vi "Periodic Tasks.vi"(8 "error in":errorcluster) -> ()   [LabVIEW 2017]
doc: "This VI runs in parallel to other tasks. It can contain as many user-defined periodic loops as you need. These can carry out PID or other sorts of timed response."
uses:
  <vilib>/Rock Robotics/WPI/DriverStation/WPI_DriverStationRobotMode2.ctl
  <vilib>/Rock Robotics/WPI/Utilities/WPI_GetSetVariantRefNum.vi
  Robot Global Data.vi
  <vilib>/Rock Robotics/WPI/RobotDrive/WPI_RobotDriveArcadeDrive_Standard(NoSaturation).vi
  <vilib>/Rock Robotics/Network Tables/NT Write Numeric Array.vi
  <vilib>/Rock Robotics/Network Tables/NT Write Number.vi
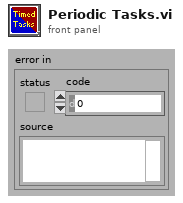
[diagram p1: front panel]
types:
  T1 = typedef "WPI_JoystickDevRef.ctl" = cluster{"Device":T2}
  T2 = typedef "WPI_JoystickDeviceEnum.ctl" = enum16{"USB 0", "USB 1", "USB 2", "USB 3", "USB 4", "USB 5"}
  T3 = typedef "WPI_RobotDriveDevRef.ctl" = cluster{"DevStatus":errorcluster, "Motors[]":T4[], "Square Inputs":bool, "Max Output":dbl}
  T4 = typedef "WPI_MotorControlDeviceRef.ctl" = cluster{"DeviceStatus":errorcluster, "Type":T5, "PWM":cluster{"PWM Channel":T6, "DeadBand":T7}, "CAN":cluster{"Device Number":u8, "SetOutput VI Ref":variant, "GetOutput VI Ref":variant, "Enable VI Ref":variant, "Disable VI Ref":variant, "Data":variant}, "Invert":bool, "DIO PWM":cluster{"PWM \"Enable\" Channel":T6, "DIOChannel":T8, "PWM Rate":dbl}}
  T5 = typedef "WPI_MotorControlType.ctl" = enum16{"PWM", "CAN", "DIO PWM"}
  T6 = typedef "FPGA_DIOPWMChannel.ctl" = enum8{"PWM 0", "PWM 1", "PWM 2", "PWM 3", "PWM 4", "PWM 5", "PWM 6", "PWM 7", "PWM 8", "PWM 9", "PWM MXP 0", "PWM MXP 1", "PWM MXP 2", "PWM MXP 3", "PWM MXP 4", "PWM MXP 5", "PWM MXP 6", "PWM MXP 7", "PWM MXP 8", "PWM MXP 9", "Invalid"}
  T7 = typedef "WPI_PWMDeadband.ctl" = cluster{"Name":string, "maxPositivePwm":i32, "minPositivePwm":i32, "centerPwm":i32, "maxNegativePwm":i32, "minNegativePwm":i32, "angularRange":u16}
  T8 = typedef "FPGA_DIOChannel.ctl" = enum8{"DIO 0", "DIO 1", "DIO 2", "DIO 3", "DIO 4", "DIO 5", "DIO 6", "DIO 7", "DIO 8", "DIO 9", "DIO MXP 0", "DIO MXP 1", "DIO MXP 2", "DIO MXP 3", "DIO MXP 4", "DIO MXP 5", "DIO MXP 6", "DIO MXP 7", "DIO MXP 8", "DIO MXP 9", "DIO MXP 10", "DIO MXP 11", "DIO MXP 12", "DIO MXP 13", "DIO MXP 14", "DIO MXP 15", "SPI Port CS1", "SPI Port CS2", "SPI Port CS3", "SPI Port MISO", "SPI Port MOSI", "Invalid"}
  T9 = cluster{"JoystickDevRef":T1, "RobotDriveDevRef":T3}
  T10 = typedef "WPI_GyroDevRef.ctl" = cluster{"DevStatus":errorcluster, "Analog Channel":T11, "Gain (VoltsPerDegree/Second)":dbl, "Gyro Type":enum16{"Analog", "XRS450"}, "Handle":i32, "SPI Bus":T12, "Device Found":bool, "Sample Rate":dbl, "Calibrate On Open":bool, "Offset":dbl}
  T11 = typedef "FPGA_AIChannel.ctl" = enum8{"AI 0", "AI 1", "AI 2", "AI 3", "AI MXP 0", "AI MXP 1", "AI MXP 2", "AI MXP 3", "Invalid"}
  T12 = typedef "spi_bus.ctl" = enum16{"SPI On-Board, CS0", "SPI On-Board, CS1", "SPI On-Board, CS2", "SPI On-Board, CS3", "SPI MXP", "Invalid"}
  T13 = typedef "WPI_DriverStationRobotMode2.ctl" = enum16{"Autonomous Disabled", "Autonomous Enabled", "Teleop Disabled", "Teleop Enabled", "Disconnected", "Finish", "Test Disabled", "Test Enabled", "Emergency Stopped"}
  T14 = typedef "WPI_CompressorDevRef.ctl" = cluster{"DevStatus":errorcluster, "Pneumatics Control Module":u8}
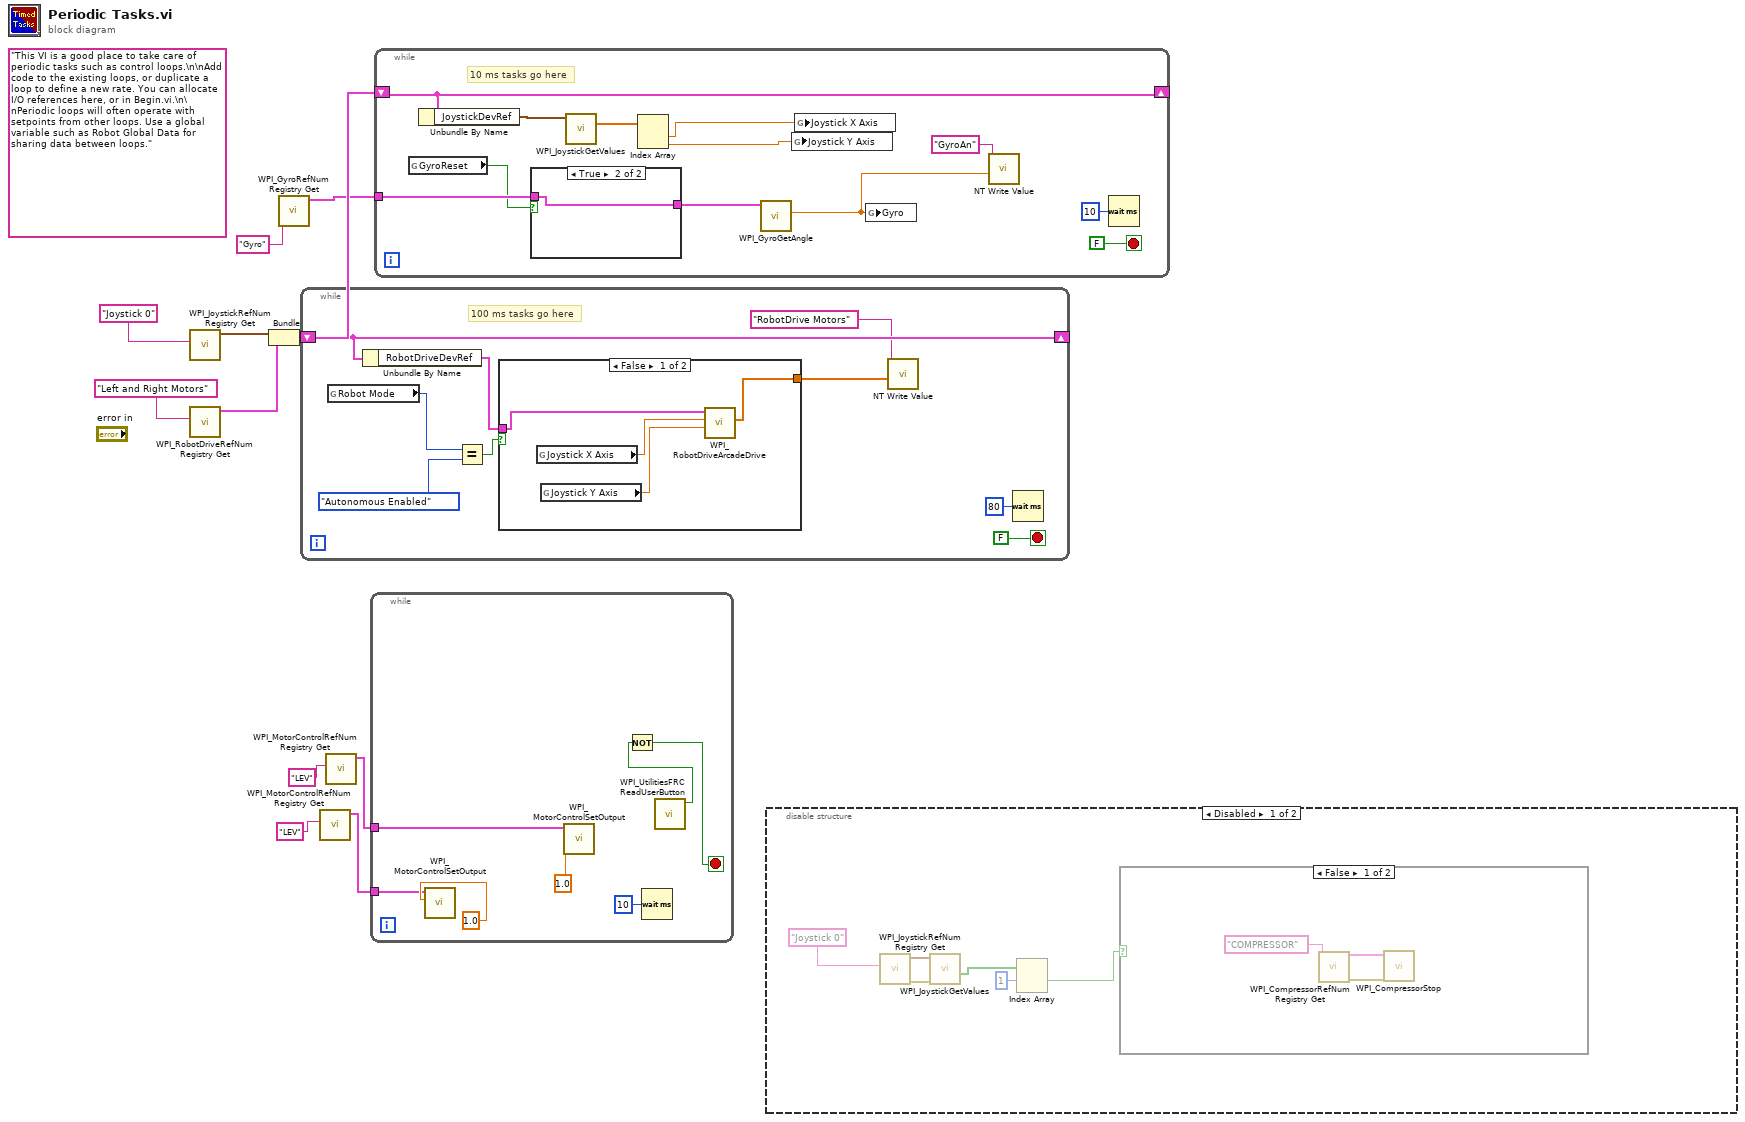
[diagram p0: block diagram]
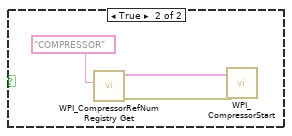
[diagram p2: hidden frame]
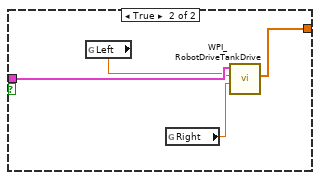
[diagram p4: hidden frame]
diagram:
  (unwired) "This VI is a good place to take care of periodic tasks such as control loops.\n\nAdd code to the existing loops, or duplicate a loop to define a new rate. You can allocate I/O references here, or in Begin.vi.\n\nPeriodic loops will often operate with setpoints from other loops. Use a global variable such as Robot Global Data for sharing data between loops."
  n1 = call <vilib>:"WPI_JoystickRefNum Registry Get.vi"("refnum name"="Joystick 0") -> ("JoystickDevRef"=w9:T1)  [unwired: 1 in, 9 out]
  n2 = call <vilib>:"WPI_RobotDriveRefNum Registry Get.vi"("refnum name"="Left and Right Motors") -> ("RobotDriveDevRef"=w8:T3)  [unwired: 1 in, 9 out]
  n3 = Bundle("JoystickDevRef"=w9, "RobotDriveDevRef"=w8) -> (w7:T9)  [unwired: 1 out]
  n4 = call <vilib>:"WPI_GyroRefNum Registry Get.vi"("refnum name"="Gyro") -> ("GyroDevRef"=w5:T10)  [unwired: 9 in, 1 out]
  n5 = while {
    shift-right: [w18] -> _
    shift-left: w7 -> [w18]
    stop <- FALSE stop-if-true
    # "100 ms tasks go here"
    n6 = global read "Robot Global Data.vi" "Robot Mode"() -> (w17:T13)
    n7 = Unbundle By Name(w18) -> ("RobotDriveDevRef"=w14:T3)
    n8 = Equal?(x=w17, y=WPI_DriverStationRobotMode2."Autonomous Enabled") -> (x = y?=w15:bool)
    n9 = case shown="False" w15 {
      tunnel: w14 -> [w24 w28]
      tunnel: [w21 w25] -> w13
      frame False {
        n10 = global read "Robot Global Data.vi" "Joystick X Axis"() -> (w23:dbl)
        n11 = global read "Robot Global Data.vi" "Joystick Y Axis"() -> (w22:dbl)
        n12 = call-poly <vilib>:"WPI_RobotDriveArcadeDrive.vi"("Y axis value"=w22, "X axis value"=w23, "RobotDriveDevRef"=w24) -> ("Motor Values"=w21:dbl[])  [unwired: 6 in, 2 out]
      }
      frame True {
        n13 = global read "Robot Global Data.vi" "Left"() -> (w26:dbl)
        n14 = global read "Robot Global Data.vi" "Right"() -> (w27:dbl)
        n15 = call <vilib>:"WPI_RobotDriveTankDrive.vi"("Right axis value"=w27, "Left axis value"=w26, "RobotDriveDevRef"=w28) -> ("Motor Values"=w25:dbl[])  [unwired: 6 in, 2 out]
      }
    }
    n16 = call-poly <vilib>:"NT Write Value.vi"("Numeric Array"=w13, "Name"="RobotDrive Motors") -> ()  [unwired: 9 in, 1 out]
    n17 = Wait (ms)(milliseconds to wait=u32 80) -> ()  [unwired: 1 out]
  }
  n18 = call <vilib>:"WPI_MotorControlRefNum Registry Get.vi"("refnum name"="LEV") -> ("MotorControlDevRef"=w1:T4)  [unwired: 9 in, 1 out]
  n19 = call <vilib>:"WPI_MotorControlRefNum Registry Get.vi"("refnum name"="LEV") -> ("MotorControlDevRef"=w2:T4)  [unwired: 9 in, 1 out]
  n20 = while {
    tunnel: w2 -> [w33]
    tunnel: w1 -> [w32]
    stop <- w29 stop-if-true
    n21 = call <vilib>:"WPI_MotorControlSetOutput.vi"("Output"=1.0, "MotorControlDevRef"=w32) -> ()  [unwired: 7 in, 3 out]
    n22 = call <vilib>:"WPI_MotorControlSetOutput.vi"("Output"=1.0, "MotorControlDevRef"=w33) -> ()  [unwired: 7 in, 3 out]
    n23 = Wait (ms)(milliseconds to wait=u32 10) -> ()  [unwired: 1 out]
    n24 = call <vilib>:"WPI_UtilitiesFRC ReadUserButton.vi"() -> ("User Button"=w30:bool)  [unwired: 10 in, 1 out]
    n25 = Not(x=w30) -> (.not. x?=w29:bool)
  }
  n26 = while {
    shift-right: [w45] -> _
    shift-left: w7 -> [w45]
    tunnel: w5 -> [w40]
    stop <- FALSE stop-if-true
    # "10 ms tasks go here"
    n27 = global read "Robot Global Data.vi" "GyroReset"() -> (w39:bool)
    n28 = Unbundle By Name(w45) -> ("JoystickDevRef"=w44:T1)
    n29 = case shown="True" w39 {
      tunnel: w40 -> [w48 w49]
      tunnel: [w48 w49] -> w38
      frame False {
      }
      frame True {
      }
    }
    n30 = call <vilib>:"WPI_JoystickGetValues.vi"("JoystickDevRef"=w44) -> ("Axes"=w43:dbl[])  [unwired: 6 in, 4 out]
    n31 = Index Array(array=w43) -> (element #1=w42:dbl, element #2=w41:dbl)  [unwired: 2 in]
    n32 = call <vilib>:"WPI_GyroGetAngle.vi"("GyroDevRef"=w38) -> ("Angle"=w37:dbl)  [unwired: 6 in, 4 out]
    n33 = global write "Robot Global Data.vi" "Joystick Y Axis"(w41) -> ()
    n34 = global write "Robot Global Data.vi" "Joystick X Axis"(w42) -> ()
    n35 = global write "Robot Global Data.vi" "Gyro"(w37) -> ()
    n36 = call-poly <vilib>:"NT Write Value.vi"("Numeric"=w37, "Name"="GyroAn") -> ()  [unwired: 9 in, 1 out]
    n37 = Wait (ms)(milliseconds to wait=u32 10) -> ()  [unwired: 1 out]
  }
  n38 = disable-structure shown="Disabled" {
    frame Disabled {
      n39 = call <vilib>:"WPI_JoystickRefNum Registry Get.vi"("refnum name"="Joystick 0") -> ("error out"=w52:errorcluster, "JoystickDevRef"=w55:T1)  [unwired: 1 in, 8 out]
      n40 = call <vilib>:"WPI_JoystickGetValues.vi"("error in (no error)"=w52, "JoystickDevRef"=w55) -> ("Buttons"=w53:bool[])  [unwired: 5 in, 4 out]
      n41 = Index Array(array=w53, index #1=1 ("index")) -> (element #1=w50:bool)  [unwired: 1 in, 1 out]
      n42 = case shown="False" w50 {
        frame False {
          n43 = call <vilib>:"WPI_CompressorRefNum Registry Get.vi"("refnum name"="COMPRESSOR") -> ("error out"=w58:errorcluster, "CompressorDevRef"=w57:T14)  [unwired: 9 in]
          n44 = call <vilib>:"WPI_CompressorStop.vi"("error in (no error)"=w58, "CompressorDevRef"=w57) -> ()  [unwired: 8 in, 2 out]
        }
        frame True {
          n45 = call <vilib>:"WPI_CompressorRefNum Registry Get.vi"("refnum name"="COMPRESSOR") -> ("error out"=w59:errorcluster, "CompressorDevRef"=w60:T14)  [unwired: 9 in]
          n46 = call <vilib>:"WPI_CompressorStart.vi"("error in (no error)"=w59, "CompressorDevRef"=w60) -> ()  [unwired: 8 in, 2 out]
        }
      }
    }
    frame Enabled {
    }
  }
